vi "Set Register Actor Message Public.vi"() -> (0 "error out":errorcluster)   [LabVIEW 2020]
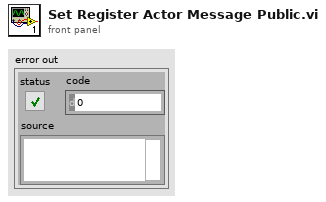
[diagram p1: front panel]
types:
  T1 = enum32{"invalid scope", "public", "private", "protected", "community"}
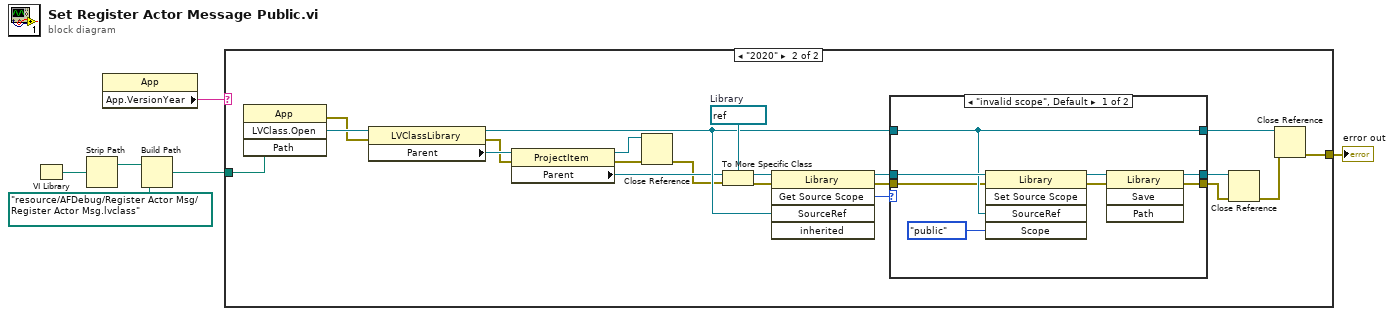
[diagram p0: block diagram]
diagram:
  n1 = VI Library() -> (path=w6:path)
  n2 = Strip Path(path=w6) -> (stripped path=w5:path)  [unwired: 1 out]
  n3 = property class="App"() -> ("App.VersionYear"=w1:string)  [unwired: 2 in, 2 out]
  n4 = Build Path(base path=w5, name or relative path=path "resource/AFDebug/Register Actor Msg/Register Actor Msg.lvclass") -> (appended path=w3:path)
  n5 = case shown="\"2020\"" w1 {
    tunnel: w3 -> [_ w27]
    tunnel: [_ w7] -> w2
    frame "False", Default {
    }
    frame "2020" {
      w25 = refnum<vi> refnum  # Library
      n6 = invoke class="App" method="LVClass.Open"("Path"=w27) -> (error out=w20:errorcluster, "LVClass.Open"=w26:refnum<vi>)  [unwired: 3 in, 2 out]
      n7 = property class="LVClassLibrary"(reference=w26, error in=w20) -> (reference out=w22:refnum<vi>, error out=w12:errorcluster, "Parent"=w13:refnum<vi>)
      n8 = property class="ProjectItem"(reference=w13, error in=w12) -> (reference out=w9:refnum<vi>, error out=w10:errorcluster, "Parent"=w11:refnum<vi>)
      n9 = Close Reference(reference=w9, error in (no error)=w10) -> (error out=w8:errorcluster)
      n10 = To More Specific Class(target class=w25, reference=w11, error in=w8) -> (specific class reference=w24:refnum<vi>, error out=w19:errorcluster)
      n11 = invoke class="Library" method="Get Source Scope"(reference=w24, error in=w19, "SourceRef"=w22) -> (reference out=w23:refnum<vi>, error out=w16:errorcluster, "GetSourceScope"=w21:T1)  [unwired: 2 in, 2 out]
      n12 = case shown="\"invalid scope\", Default" w21 {
        tunnel: w23 -> [w35 w37]
        tunnel: w22 -> [w33 w38]
        tunnel: [w33 w38] -> w17
        tunnel: [w29 w37] -> w18
        tunnel: w16 -> [w32 w36]
        tunnel: [w28 w36] -> w15
        frame "invalid scope", Default {
          n13 = invoke class="Library" method="Set Source Scope"(reference=w35, error in=w32, "SourceRef"=w33, "Scope"=T1."public" ("scope")) -> (reference out=w31:refnum<vi>, error out=w30:errorcluster)  [unwired: 1 in, 3 out]
          n14 = invoke class="Library" method="Save"(reference=w31, error in=w30) -> (reference out=w29:refnum<vi>, error out=w28:errorcluster)  [unwired: 2 in, 2 out]
        }
        frame "public" {
        }
      }
      n15 = Close Reference(reference=w18, error in (no error)=w15) -> (error out=w14:errorcluster)
      n16 = Close Reference(reference=w17, error in (no error)=w14) -> (error out=w7:errorcluster)
    }
  }
  "error out" <- w2
